vi "Login GUI.vi"() -> (3 "true":bool)   [LabVIEW 2017]
uses:
  admin_settings.vi
panel:
  in  "Cancel":bool
  in  "Accept":bool
  in  "Password":string
  in  "User":string
  # "Sign in"
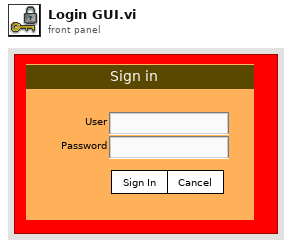
[diagram p1: front panel]
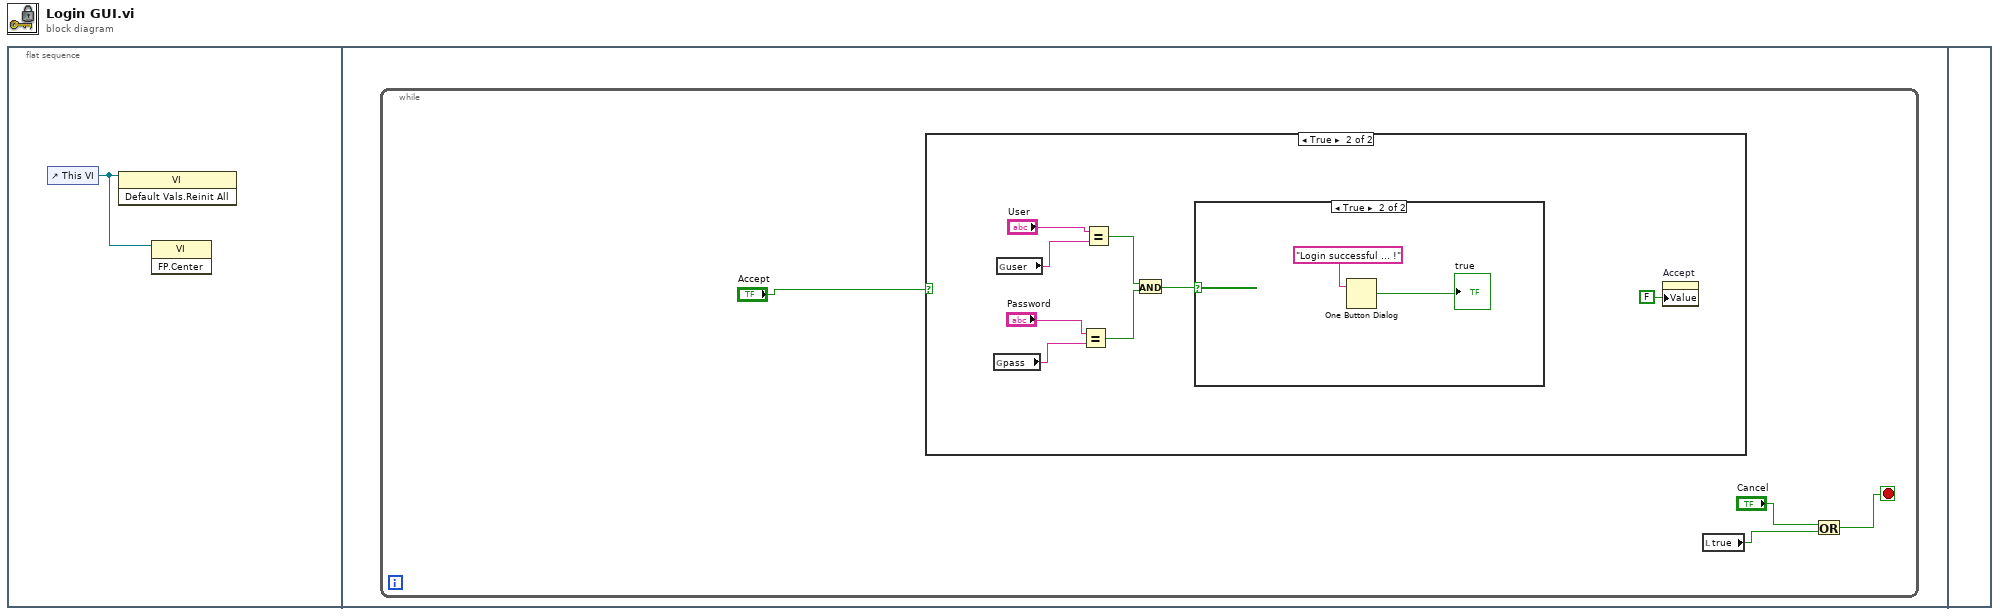
[diagram p0: block diagram]
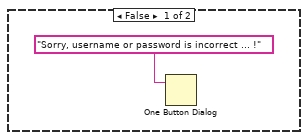
[diagram p3: hidden frame]
diagram:
  n1 = flat-sequence {
    frame #0 {
      n2 = control-ref of="This VI"() -> (w1:refnum<vi>)
      n3 = invoke class="VI" method="Default Vals.Reinit All"(reference=w1) -> ()  [unwired: 2 in, 3 out]
      n4 = invoke class="VI" method="FP.Center"(reference=w1) -> ()  [unwired: 2 in, 3 out]
    }
    frame #1 {
      n5 = while {
        stop <- w3 stop-if-true
        n6 = case shown="True" "Accept" {
          frame False {
          }
          frame True {
            n7 = global read "admin_settings.vi" "pass"() -> (w10:string)
            n8 = global read "admin_settings.vi" "user"() -> (w12:string)
            n9 = Equal?(x="Password", y=w10) -> (x = y?=w8:bool)
            n10 = Equal?(x="User", y=w12) -> (x = y?=w9:bool)
            n11 = And(x=w9, y=w8) -> (x .and. y?=w7:bool)
            n12 = case shown="True" w7 {
              frame False {
                n13 = One Button Dialog(message="Sorry, username or password is incorrect ... !") -> ()  [unwired: 1 in, 1 out]
              }
              frame True {
                n14 = One Button Dialog(message="Login successful ... !") -> (true=→"true":bool)  [unwired: 1 in]
              }
            }
            n15 = property on="Accept" class="Bool (strict)"("Value"=FALSE ("Accept")) -> ()  [unwired: 2 in, 2 out]
          }
        }
        n16 = local read "true"() -> (w2:bool)
        n17 = Or(x="Cancel", y=w2) -> (x .or. y?=w3:bool)
      }
    }
    frame #2 {
    }
  }
